vi "Size Selector.vi"   [LabVIEW 2020, in "Panel.lvlib"]
doc: "Polymorphic VI to select an appropriate Size Selector.\n\n----\nPlease see the following web address for additional documentation and tutorial information:\nhttp://www.mooregoodideas.com/mgi-panel-manager/\n\nAuthor: Derek Trepanier\n\nCopyright (c) 2018, Moore Good Ideas, Inc.\n\nAll rights reserved.\n\nRedistribution and use in source and binary forms, with or without modification, are permitted provided that the following conditions are met:\n\n * Redistributions of source code must retain the above copyright notice, this list of conditions and the following disclaimer.\n * Redistributions in binary form must reproduce the above copyright notice, this list of conditions and the following disclaimer in the documentation and/or other materials provided with the distribution.\n * Neither the name of Moore Good Ideas, Inc. nor the names of its contributors may be used to endorse or promote products derived from this software without specific prior written permission.\n\nTHIS SOFTWARE IS PROVIDED BY THE COPYRIGHT HOLDERS AND CONTRIBUTORS \"AS IS\" AND ANY EXPRESS OR IMPLIED WARRANTIES, INCLUDING, BUT NOT LIMITED TO, THE IMPLIED WARRANTIES OF MERCHANTABILITY AND FITNESS FOR A PARTICULAR PURPOSE ARE DISCLAIMED. IN NO EVENT SHALL THE COPYRIGHT OWNER OR CONTRIBUTORS BE LIABLE FOR ANY DIRECT, INDIRECT, INCIDENTAL, SPECIAL, EXEMPLARY, OR CONSEQUENTIAL DAMAGES (INCLUDING, BUT NOT LIMITED TO, PROCUREMENT OF SUBSTITUTE GOODS OR SERVICES; LOSS OF USE, DATA, OR PROFITS; OR BUSINESS INTERRUPTION) HOWEVER CAUSED AND ON ANY THEORY OF LIABILITY, WHETHER IN CONTRACT, STRICT LIABILITY, OR TORT (INCLUDING NEGLIGENCE OR OTHERWISE) ARISING IN ANY WAY OUT OF THE USE OF THIS SOFTWARE, EVEN IF ADVISED OF THE POSSIBILITY OF SUCH DAMAGE."
uses:
  <vilib>/MGI/Panel Manager/Panel/Panel.lvlib
  <vilib>/MGI/Panel Manager/Panel/Window Position/Reference Position/Size/Absolute Size/Absolute Size.lvclass
  <vilib>/MGI/Panel Manager/Panel/Window Position/Reference Position/Size/Reference Size/Reference Size.lvclass
  <vilib>/MGI/Panel Manager/Panel/Window Position/Reference Position/Size/Auto-Stretch/Auto-Stretch.lvclass
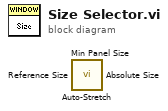
[diagram p0: block diagram]
diagram:
  n1 = call <vilib>:"Auto-Stretch.vi"() -> ()  [unwired: 10 in, 2 out]
  n2 = call <vilib>:"Min Panel Size.vi"() -> ()  [unwired: 10 in, 2 out]
  n3 = call <vilib>:"Reference Size.vi"() -> ()  [unwired: 10 in, 2 out]
  n4 = call <vilib>:"Absolute Size.vi"() -> ()  [unwired: 10 in, 2 out]
